vi "Parse Lights JSON.vi"(8 "Error In":errorcluster, 10 "Light JSON":string="{\"1\":{\"name\": \"Hue Lamp\"},\"2\":{\"name\": \"Hue Lamp 1\"},\"3\":{\"name\": \"Hue Lamp 2\"}}") -> (0 "Error Out":errorcluster, 2 "Lights":T1[](array[typedef]))   [LabVIEW 2013, in "LVH-Hue.lvlib"]
uses:
  LVH-Hue.lvlib
  Type Defs/Light.ctl
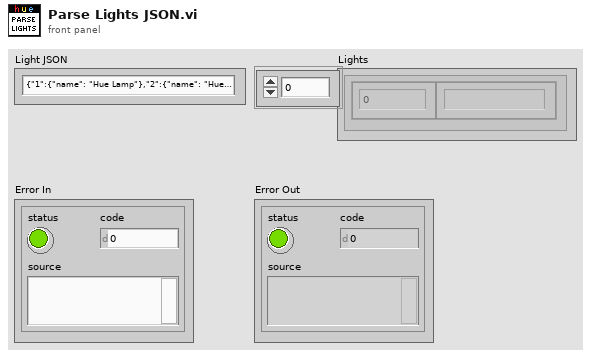
[diagram p1: front panel]
types:
  T1 = typedef "LVH-Hue.lvlib/Light.ctl" = cluster{"ID":i32, "Name":string}
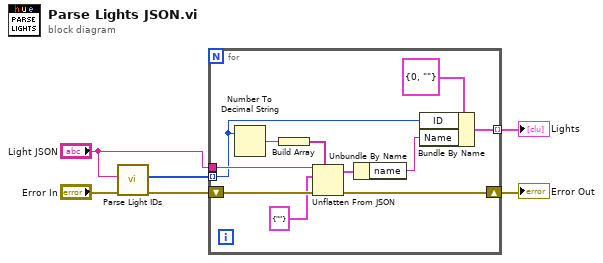
[diagram p0: block diagram]
diagram:
  n1 = call "Parse Light IDs.vi"("Error In"="Error In", "Light JSON"="Light JSON") -> ("Error Out"=w5:errorcluster, "Light IDs"=w4:i32[])  [unwired: 8 in]
  n2 = for {
    tunnel: w4 -> [w13] mode=indexing
    tunnel: "Light JSON" -> [w16]
    tunnel: [w10] -> w2 mode=indexing
    shift-right: [w9] -> w1
    shift-left: w5 -> [w17]
    n3 = Number To Decimal String(number=w13) -> (decimal integer string=w8:string)  [unwired: 1 in]
    n4 = Build Array(w8) -> (w7:string[])
    n5 = Unflatten From JSON(path=w7, JSON string=w16, type and defaults=cluster{"name":string} {"name"=""}, error in (no error)=w17) -> (value=w12:cluster{"name":string}, error out=w9:errorcluster)  [unwired: 3 in]
    n6 = Unbundle By Name(w12) -> ("name"=w11:string)
    n7 = Bundle By Name(cluster=T1 {"ID"=0, "Name"=""} ("Light"), "ID"=w13, "Name"=w11) -> (w10:T1)
  }
  "Error Out" <- w1
  "Lights" <- w2
